vi "Scope Report Event.vi"(8 "error in (no error)":errorcluster, 9 "Event Data":variant, 10 "Scope Events":T1, 11 "Controller in":refnum<class "Controller.lvclass">) -> (0 "error out":errorcluster, 3 "Controller out":refnum<class "Controller.lvclass">)   [LabVIEW 2020, in "Controller.lvlib" / "Controller.lvclass"]
uses:
  Controller.lvclass
  C:/Program Files/National Instruments/LabVIEW 2020/vi.lib/ActorFramework/Actor/Actor.lvclass
  Actor_Scope/Actor_Scope/Scope_Event.ctl
  <vilib>/ActorFramework/Actor/Actor.lvclass/Actor.ctl
  <vilib>/ActorFramework/Message Enqueuer/Message Enqueuer.lvclass/Message Enqueuer.ctl
  Controller.lvclass/Controller.ctl
  Actor_log/Actor_log Messages/Write Event to Log Msg/Write Event to Log Msg.lvclass/Write Event to Log Msg.ctl
  Actor_AFG/Actor_AFG Messages/AFG Enable Output Msg/AFG Enable Output Msg.lvclass/AFG Enable Output Msg.ctl
  <vilib>/Analysis/baseanly.llb/Mean (DBL).vi
  <vilib>/ActorFramework/Message Enqueuer/Init from Existing Queue.vi
  <vilib>/ActorFramework/Stop Msg/Send Emergency Stop.vi
  <vilib>/ActorFramework/Stop Msg/Send Normal Stop.vi
  <vilib>/ActorFramework/Message Enqueuer/Enqueue.vi
  <vilib>/ActorFramework/Message Enqueuer/Enqueue Critical.vi
  <vilib>/ActorFramework/Stop Msg/Stop Msg.lvclass
  C:/Program Files/National Instruments/LabVIEW 2020/vi.lib/ActorFramework/Message/Message.lvclass
  Actor_log/Actor_log Messages/Write Event to Log Msg/Write Event to Log Msg.lvclass
  Actor_AFG/Actor_AFG Messages/AFG Enable Output Msg/AFG Enable Output Msg.lvclass
  <vilib>/ActorFramework/Message Priority Queue/Priority Enqueue.vi
  <vilib>/measure/mascope.llb/Amplitude and Levels 1 chan.vi
  <vilib>/ActorFramework/Message Enqueuer/Message Enqueuer.lvclass
  <vilib>/ActorFramework/Actor/Actor.lvclass
  <vilib>/measure/NI_MAPro.lvlib
  <vilib>/Analysis/NI_AALBase.lvlib
  Actor_Scope/Actor_Scope/Actor_Scope.lvclass
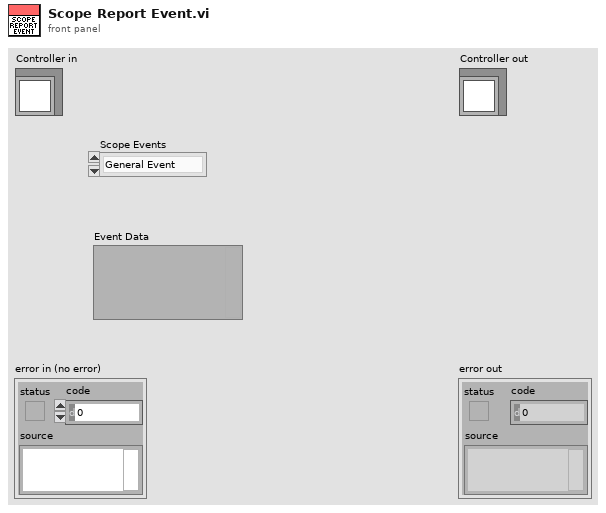
[diagram p1: front panel]
types:
  T1 = typedef "Actor_Scope.lvlib/Actor_Scope.lvclass/Scope_Event.ctl" = enum16{"General Event", "Inited", "Error", "Res Read complete", "Wfm Acq Complete"}
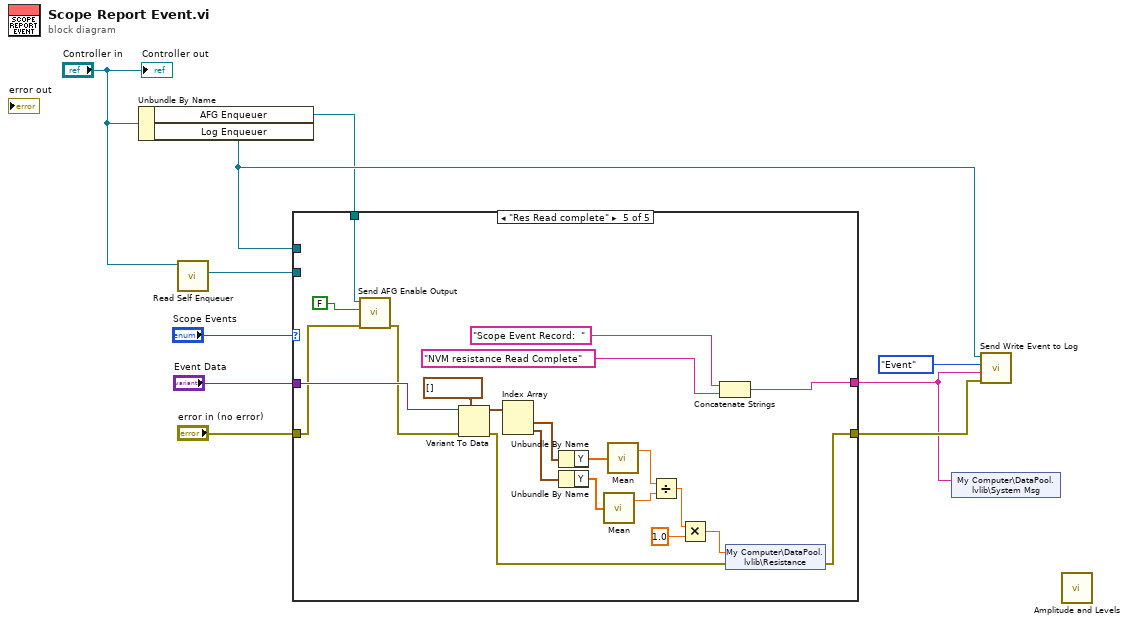
[diagram p0: block diagram]
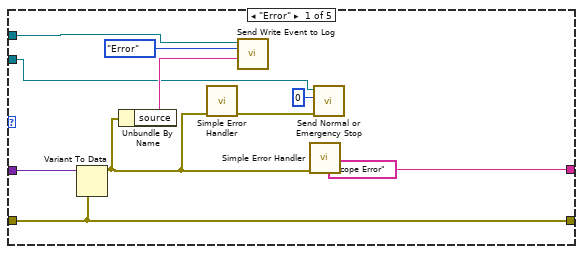
[diagram p2: hidden frame]
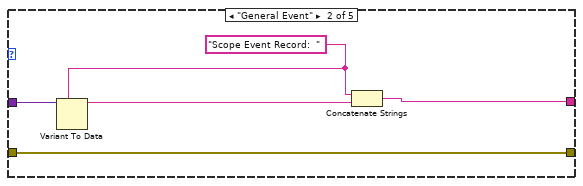
[diagram p3: hidden frame]
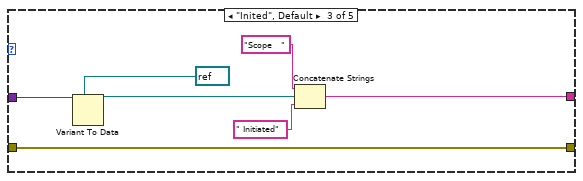
[diagram p4: hidden frame]
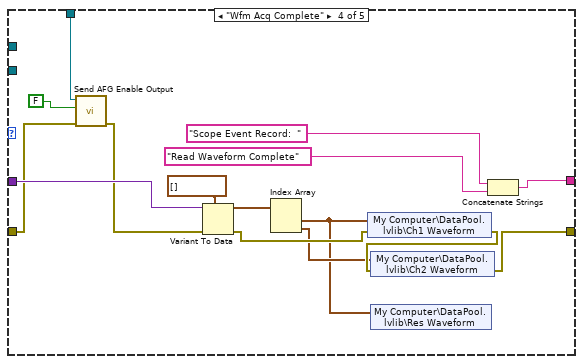
[diagram p5: hidden frame]
diagram:
  n1 = Unbundle By Name("Controller in") -> ("AFG Enqueuer"=w2:refnum<class "Message Enqueuer.lvclass">, "Log Enqueuer"=w4:refnum<class "Message Enqueuer.lvclass">)
  n2 = call <vilib>:"Read Self Enqueuer.vi"("Actor"="Controller in") -> ("Self Enqueuer"=w6:refnum<class "Message Enqueuer.lvclass">)  [unwired: 10 in]
  n3 = case shown="\"Res Read complete\"" "Scope Events" {
    tunnel: "Event Data" -> [w19 w23 w32 w44 w65]
    tunnel: "error in (no error)" -> [w20 w25 w27 w35 w60]
    tunnel: [w20 w25 w27 w39 w48] -> w3
    tunnel: ["Scope Error" w21 w26 w45 w66] -> w1
    tunnel: w6 -> [w11 _ _ _ _]
    tunnel: w4 -> [w16 _ _ _ _]
    tunnel: w2 -> [_ _ _ w37 w62]
    frame "Error" {
      n4 = Variant To Data(type=w20, Variant=w19) -> (data=w12:errorcluster)  [unwired: 1 in, 1 out]
      n5 = Unbundle By Name(w12) -> ("source"=w15:string)
      n6 = call <vilib>:"Simple Error Handler.vi"("error in (no error)"=w12) -> ("error out"=w14:errorcluster)  [unwired: 4 in, 4 out]
      n7 = call "Send Write Event to Log.vi"("Log Event Details"=w15, "Enum"=enum16{"Event", "Error"}."Error", "Message Enqueuer"=w16) -> ()  [unwired: 7 in, 2 out]
      n8 = call <vilib>:"Simple Error Handler.vi"("error in (no error)"=w12) -> ()  [unwired: 4 in, 5 out]
      n9 = call <vilib>:"Send Normal or Emergency Stop.vi"("error in (no error)"=w14, "final error code"=0, "Message Enqueuer"=w11) -> ()  [unwired: 8 in, 1 out]
    }
    frame "General Event" {
      w24 = "Scope Event Record:  "
      n10 = Variant To Data(type=w24, Variant=w23) -> (data=w22:string)  [unwired: 1 in, 1 out]
      n11 = Concatenate Strings(w24, w22) -> (w21:string)
    }
    frame "Inited", Default {
      n12 = Variant To Data(type=refnum<visa-resource-name> refnum ("VISA resource name"), Variant=w32) -> (data=w30:refnum<visa-resource-name>)  [unwired: 1 in, 1 out]
      n13 = Concatenate Strings("Scope   " ("string"), w30, " Initiated" ("string")) -> (w26:string)
    }
    frame "Wfm Acq Complete" {
      n14 = call "Send AFG Enable Output.vi"("error in (no error)"=w35, "Enable Output (T: Enable)"=FALSE, "Message Enqueuer"=w37) -> ("error out"=w34:errorcluster)  [unwired: 7 in, 1 out]
      n15 = Variant To Data(error in=w34, type=waveform(dbl)[] [], Variant=w44) -> (data=w42:waveform(dbl)[], error out=w41:errorcluster)
      n16 = Index Array(array=w42) -> (element #1=w33:waveform(dbl), element #2=w38:waveform(dbl))  [unwired: 2 in]
      n17 = shared-variable "My Computer\\DataPool.lvlib\\Ch1 Waveform"(w33, error in=w41) -> (error out=w40:errorcluster)
      n18 = shared-variable "My Computer\\DataPool.lvlib\\Ch2 Waveform"(w38, error in=w40) -> (error out=w39:errorcluster)
      n19 = shared-variable "My Computer\\DataPool.lvlib\\Res Waveform"(w33) -> ()  [unwired: 1 in, 1 out]
      n20 = Concatenate Strings("Scope Event Record:  ", "Read Waveform Complete" ("string")) -> (w45:string)
    }
    frame "Res Read complete" {
      n21 = call "Send AFG Enable Output.vi"("error in (no error)"=w60, "Enable Output (T: Enable)"=FALSE, "Message Enqueuer"=w62) -> ("error out"=w59:errorcluster)  [unwired: 7 in, 1 out]
      n22 = Variant To Data(error in=w59, type=waveform(dbl)[] [], Variant=w65) -> (data=w63:waveform(dbl)[], error out=w49:errorcluster)
      n23 = Index Array(array=w63) -> (element #1=w58:waveform(dbl), element #2=w57:waveform(dbl))  [unwired: 2 in]
      n24 = Unbundle By Name(w58) -> ("Y"=w56:dbl[])
      n25 = Unbundle By Name(w57) -> ("Y"=w55:dbl[])
      n26 = call-poly <vilib>:"Mean.vi"("X"=w55) -> ("mean"=w53:dbl)  [unwired: 1 out]
      n27 = call-poly <vilib>:"Mean.vi"("X"=w56) -> ("mean"=w54:dbl)  [unwired: 1 out]
      n28 = Divide(x=w54, y=w53) -> (x/y=w52:dbl)
      n29 = Multiply(x=w52, y=1.0) -> (x*y=w50:dbl)
      n30 = Concatenate Strings("Scope Event Record:  ", "NVM resistance Read Complete" ("string")) -> (w66:string)
      n31 = shared-variable "My Computer\\DataPool.lvlib\\Resistance"(w50, error in=w49) -> (error out=w48:errorcluster)
    }
  }
  n32 = shared-variable "My Computer\\DataPool.lvlib\\System Msg"(w1) -> ()  [unwired: 1 in, 1 out]
  n33 = call "Send Write Event to Log.vi"("error in (no error)"=w3, "Log Event Details"=w1, "Enum"=enum16{"Event", "Error"}."Event", "Message Enqueuer"=w4) -> ()  [unwired: 6 in, 2 out]
  n34 = call-poly <vilib>:"Amplitude and Levels.vi"() -> ()  [unwired: 8 in, 4 out]
  "Controller out" <- "Controller in"
